vi "HFRR ADV v026 new software.vi"() -> ()   [LabVIEW 2025] (continued)
        n1473 = property on="Dashboard" class="Bool (strict)"("DisabledEnum"=w1348) -> ()  [unwired: 2 in, 2 out]
        n1474 = property on="Analysis" class="Bool (strict)"("DisabledEnum"=w1348) -> ()  [unwired: 2 in, 2 out]
        n1475 = property on="Home" class="Bool (strict)"("DisabledEnum"=w1348) -> ()  [unwired: 2 in, 2 out]
        n1476 = property on="Report" class="Bool (strict)"("DisabledEnum"=w1348) -> ()  [unwired: 2 in, 2 out]
        n1477 = property on="Calibration" class="Bool (strict)"("DisabledEnum"=w1348) -> ()  [unwired: 2 in, 2 out]
      }
      frame "About" {
        n1478 = local read "FILE"() -> (w1367:string)
        n1479 = local read "TEST FILE NAM,E SAVED"() -> (w1360:bool)
        n1480 = call <vilib>:"Trim Whitespace.vi"("string"=w1367) -> ("trimmed string"=w1366:string)  [unwired: 1 in]
        n1481 = local read "Auto Start Test"() -> (w1370:bool)
        n1482 = String Length(string=w1366) -> (length=w1365:i32)
        n1483 = Greater?(x=w1365, y=1) -> (0:w1362:bool)
        n1484 = And(x=w1362, y=w1360) -> (x .and. y?=w1361:bool)
        n1485 = local read "RUN"() -> (w1372:bool)
        n1486 = case shown="True" w1361 {
          tunnel: [T18."Disabled" ("Disabled") T18."Enabled" ("Disabled")] -> w1363
          frame False {
          }
          frame True {
          }
        }
        n1487 = Or(x=w1372, y=w1370) -> (x .or. y?=w1371:bool)
        n1488 = property on="About" class="Bool (strict)"("DisabledEnum"=T18."Enabled" ("Disabled")) -> ()  [unwired: 2 in, 2 out]
        n1489 = case shown="False" w1371 {
          tunnel: [T18."Enabled" ("Disabled") T18."Disabled" ("Disabled")] -> w1369
          frame False {
          }
          frame True {
          }
        }
        n1490 = property on="Dashboard" class="Bool (strict)"("DisabledEnum"=w1363) -> ()  [unwired: 2 in, 2 out]
        n1491 = property on="Test Setup" class="Bool (strict)"("DisabledEnum"=T18."Disabled" ("Disabled")) -> ()  [unwired: 2 in, 2 out]
        n1492 = property on="Imaging" class="Bool (strict)"("DisabledEnum"=w1369) -> ()  [unwired: 2 in, 2 out]
        n1493 = property on="Analysis" class="Bool (strict)"("DisabledEnum"=w1369) -> ()  [unwired: 2 in, 2 out]
        n1494 = property on="Home" class="Bool (strict)"("DisabledEnum"=w1369) -> ()  [unwired: 2 in, 2 out]
        n1495 = property on="Report" class="Bool (strict)"("DisabledEnum"=w1369) -> ()  [unwired: 2 in, 2 out]
      }
    }
    n1496 = local read "Quit"() -> (w1297:bool)
    "Single" <- "Single - Graph"
  }
  n1497 = disable-structure shown="Disabled" {
    disable-tunnel: [w1649 _] -> w42
    disable-tunnel: _ -> [w1648 _]
    frame Disabled {
      n1498 = while {
        tunnel: w1648 -> [_]
        tunnel: [w1650] -> w1649
        tunnel: [w1651] -> _
        i -> [w1651]
        stop <- w1650 stop-if-true
        w1667 = u16 10 items=["1.0"=10, "1.5"=15, "2.0"=20] ("stop bits (10: 1 bit)")
        n1499 = Wait (ms)(milliseconds to wait=u32 10) -> ()  [unwired: 1 out]
        n1500 = call-poly "VISA Configure Serial Port"("VISA resource name"=refnum<visa-resource-name> "ASRL1::INSTR" ("COM PORT"), "timeout (10sec)"=u32 10, "baud rate (9600)"=u32 57600, "data bits (8)"=u16 8, "stop bits (10: 1 bit)"=w1667) -> ("VISA resource name out"=w1653:refnum<visa-resource-name>, "error out"=w1662:errorcluster)  [unwired: 9 in]
        n1501 = VISA Read(VISA resource name=w1653, byte count=u32 2 ("byte count (0)")) -> (read buffer=w1661:string)  [unwired: 1 in, 3 out]
        n1502 = String Subset(string=w1661, offset (0)=0, length (rest)=2 ("length (rest)")) -> (substring=w1660:string)
        n1503 = Match Pattern(string=w1660, regular expression="<>") -> (offset past match=w1657:i32)  [unwired: 1 in, 3 out]
        n1504 = Greater Or Equal?(x=w1657, y=0) -> (x >= y?=w1652:bool)
        n1505 = case shown="True" w1652 {
          tunnel: w1653 -> [_ w1671]
          tunnel: w1662 -> [_ w1670]
          frame False {
          }
          frame True {
            n1506 = VISA Read(VISA resource name=w1671, byte count=u32 32 ("byte count (0)"), error in (no error)=w1670) -> (read buffer=w1669:string)  [unwired: 3 out]
            n1507 = String Subset(string=w1669, offset (0)=0, length (rest)=8 ("length (rest)")) -> (substring=w1673:string)
            n1508 = String Subset(string=w1669, offset (0)=8, length (rest)=8 ("length (rest)")) -> (substring=w1674:string)
            n1509 = Decimal String To Number(string=w1674) -> (number=w1681:i32)  [unwired: 2 in, 1 out]
            n1510 = Decimal String To Number(string=w1673) -> (number=w1677:i32)  [unwired: 2 in, 1 out]
            n1511 = Divide(x=w1681, y=10000) -> ()  [unwired: 1 out]
            n1512 = Divide(x=w1677, y=1000000) -> ()  [unwired: 1 out]
          }
        }
        n1513 = local read "Quit"() -> (w1650:bool)
      }
    }
    frame Enabled {
    }
  }
  n1514 = Tick Count (ms)() -> (millisecond timer value=w4:u32)
  n1515 = while {
    shift-right: [w1727] -> _
    shift-left: w6 -> [w1731]
    shift-right: [w1726] -> _
    shift-left: w5 -> [w1730]
    shift-right: [w1725] -> _
    shift-left: w6 -> [w1729]
    shift-right: [w1724] -> _
    shift-left: w5 -> [w1728]
    shift-right: [w1722] -> _
    shift-left: w4 -> [w1723]
    shift-right: [w1719] -> _
    shift-left: w3 -> [w1720]
    shift-right: [w1718] -> _
    shift-left: w3 -> [w1721]
    shift-right: [w1711] -> _
    shift-left: w3 -> [w1717]
    shift-right: [w1710] -> _
    shift-left: w3 -> [w1716]
    shift-right: [w1709] -> _
    shift-left: w3 -> [w1715]
    shift-right: [w1708] -> _
    shift-left: w3 -> [w1714]
    shift-right: [w1707] -> _
    shift-left: w3 -> [w1713]
    shift-right: [w1706] -> _
    shift-left: w3 -> [w1712]
    shift-right: [w1705] -> _
    shift-left: w3 -> [w1699]
    shift-right: [w1704] -> _
    shift-left: w3 -> [w1698]
    shift-right: [w1703] -> _
    shift-left: w3 -> [w1697]
    shift-right: [w1702] -> _
    shift-left: w3 -> [w1696]
    shift-right: [w1701] -> _
    shift-left: w3 -> [w1695]
    shift-right: [w1700] -> _
    shift-left: w3 -> [w1694]
    shift-right: [w1685] -> _
    shift-left: w3 -> [w1688]
    shift-right: [w1684] -> _
    shift-left: w3 -> [w1687]
    shift-right: [w1683] -> _
    shift-left: w3 -> [w1686]
    stop <- w1733 stop-if-true
    n1516 = local read "Read UNO"() -> (w1692:string)
    n1517 = local read "Error  2"() -> (w1732:errorcluster)
    n1518 = String Length(string=w1692) -> (length=w1691:i32)
    n1519 = call <vilib>:"Trim Whitespace.vi"("string"=w1692) -> ("trimmed string"=w1693:string)  [unwired: 1 in]
    n1520 = Greater Or Equal?(x=w1691, y=23) -> (x >= y?=w1689:bool)
    n1521 = case shown="No Error" w1732 {
      tunnel: w1731 -> [w1779 w1875]
      tunnel: w1730 -> [w1778 w1874]
      tunnel: w1729 -> [w1777 w1873]
      tunnel: w1728 -> [w1776 w1872]
      tunnel: [w1775 w1875] -> w1727
      tunnel: [w1774 w1874] -> w1726
      tunnel: [w1773 w1873] -> w1725
      tunnel: [w1772 w1872] -> w1724
      tunnel: w1723 -> [w1771 w1871]
      tunnel: [w1770 w1871] -> w1722
      tunnel: w1720 -> [w1769 w1870]
      tunnel: w1721 -> [w1768 w1869]
      tunnel: [w1767 w1870] -> w1719
      tunnel: [w1766 w1869] -> w1718
      tunnel: w1717 -> [w1765 w1868]
      tunnel: w1716 -> [w1764 w1867]
      tunnel: w1715 -> [w1763 w1866]
      tunnel: w1714 -> [w1762 w1865]
      tunnel: w1713 -> [w1761 w1864]
      tunnel: w1712 -> [w1760 w1863]
      tunnel: [w1759 w1868] -> w1711
      tunnel: [w1758 w1867] -> w1710
      tunnel: [w1757 w1866] -> w1709
      tunnel: [w1756 w1865] -> w1708
      tunnel: [w1755 w1864] -> w1707
      tunnel: [w1754 w1863] -> w1706
      tunnel: w1699 -> [w1753 w1862]
      tunnel: [w1752 w1862] -> w1705
      tunnel: [w1751 w1858] -> w1704
      tunnel: [w1750 w1857] -> w1703
      tunnel: [w1749 w1861] -> w1702
      tunnel: [w1748 w1860] -> w1701
      tunnel: [w1747 w1859] -> w1700
      tunnel: w1698 -> [w1746 w1861]
      tunnel: w1697 -> [w1745 w1860]
      tunnel: w1696 -> [w1744 w1859]
      tunnel: w1695 -> [w1743 w1858]
      tunnel: w1694 -> [w1742 w1857]
      tunnel: w1693 -> [w1741 _]
      tunnel: w1689 -> [w1740 _]
      tunnel: w1688 -> [w1739 w1856]
      tunnel: w1687 -> [w1738 w1855]
      tunnel: w1686 -> [w1737 w1854]
      tunnel: [w1736 w1856] -> w1685
      tunnel: [w1735 w1855] -> w1684
      tunnel: [w1734 w1854] -> w1683
      frame No Error {
        n1522 = case shown="True" w1740 {
          tunnel: w1779 -> [w1795 w1847]
          tunnel: w1778 -> [w1794 w1846]
          tunnel: w1777 -> [w1793 w1845]
          tunnel: w1776 -> [w1792 w1844]
          tunnel: [w1795 w1843] -> w1775
          tunnel: [w1794 w1842] -> w1774
          tunnel: [w1793 w1841] -> w1773
          tunnel: [w1792 w1840] -> w1772
          tunnel: w1771 -> [w1791 w1838]
          tunnel: [w1791 w1837] -> w1770
          tunnel: w1769 -> [w1790 w1836]
          tunnel: w1768 -> [w1789 w1835]
          tunnel: [w1790 w1834] -> w1767
          tunnel: [w1789 w1833] -> w1766
          tunnel: w1765 -> [w1788 w1832]
          tunnel: w1764 -> [w1787 w1831]
          tunnel: w1763 -> [w1786 w1830]
          tunnel: w1762 -> [w1785 w1829]
          tunnel: w1761 -> [w1784 w1828]
          tunnel: w1760 -> [w1783 w1827]
          tunnel: [w1788 w1826] -> w1759
          tunnel: [w1787 w1825] -> w1758
          tunnel: [w1786 w1824] -> w1757
          tunnel: [w1785 w1823] -> w1756
          tunnel: [w1784 w1822] -> w1755
          tunnel: [w1783 w1821] -> w1754
          tunnel: w1753 -> [w1801 w1820]
          tunnel: [w1801 w1819] -> w1752
          tunnel: [w1798 w1818] -> w1751
          tunnel: [w1797 w1817] -> w1750
          tunnel: [w1800 w1816] -> w1749
          tunnel: [w1796 w1815] -> w1748
          tunnel: [w1799 w1814] -> w1747
          tunnel: w1746 -> [w1800 w1813]
          tunnel: w1745 -> [w1799 w1812]
          tunnel: w1744 -> [w1798 w1811]
          tunnel: w1743 -> [w1797 w1810]
          tunnel: w1742 -> [w1796 w1809]
          tunnel: w1741 -> [_ w1808]
          tunnel: w1739 -> [w1782 w1807]
          tunnel: w1738 -> [w1781 w1806]
          tunnel: w1737 -> [w1780 w1805]
          tunnel: [w1782 w1804] -> w1736
          tunnel: [w1781 w1803] -> w1735
          tunnel: [w1780 w1802] -> w1734
          frame False {
          }
          frame True {
            n1523 = Tick Count (ms)() -> (millisecond timer value=w1839:u32)
            n1524 = String To Byte Array(string=w1808) -> (unsigned byte array=w1852:u8[])
            n1525 = Array Size(array=w1852) -> (size(s)=w1851:i32)
            n1526 = formula code="// --- INTERNAL VARIABLE DECLARATIONS ---\nint i = 0;\nint k = 0;\nint start_idx = -1;\nint end_idx = -1;\nint phase = 0;\nint sign0 = 1;\nint sign1 = 1;\nint ch0_val = 0;   \nint ch1_val = 0;   \nfloat ch0_raw = 0.0;\nfloat ch1_raw = 0.0;\nfloat temp0 = 0.0;\nfloat temp1 = 0.0;\nfloat ch0_clean = 0.0;\nfloat ch1_clean = 0.0;\n\n// Temporal intermediate variables for calculation smoothing\nfloat raw_p2p_v = 0.0;\nfloat raw_friction = 0.0;\nfloat raw_cof = 0.0;\n\n// Initialize output variables to current shift register states right away\nout_LVDT_Min_V = in_LVDT_Min_V;\nout_LVDT_Max_V = in_LVDT_Max_V;\nout_LVDT_P2P_V = in_LVDT_P2P_V;\nout_Piezo_P2P = in_Piezo_P2P;\nout_Friction_N = in_Friction_N;\nout_COF = in_COF;\nwindow_ready = 0;\n\n// --- STEP 1: PARSE EVERY STRING IN THE BYTE ARRAY ---\nif (array_size > 2) {\n    for (i = 0; i < array_size - 1; i++) {\n        if (raw_bytes[i] == 42) { // '*' character detected\n            start_idx = i;\n        }\n        \n        // Match standard delimiter sequence \";&\" or end window character\n        if (raw_bytes[i] == 59 && raw_bytes[i+1] == 38 && start_idx != -1) { \n            end_idx = i;\n            ch0_val = 0;\n            ch1_val = 0;\n            sign0 = 1;\n            sign1 = 1;\n            phase = 0; \n\n            for (k = start_idx + 1; k < end_idx; k++) {\n                if (raw_bytes[k] == 45) { // '-' sign\n                    if (phase == 0) sign0 = -1;\n                    else sign1 = -1;\n                }\n                else if (raw_bytes[k] == 43) { // '+' sign\n                    if (phase == 0) sign0 = 1;\n                    else sign1 = 1;\n                }\n                else if (raw_bytes[k] == 59) { // ';' delimiter\n                    phase = 1; \n                }\n                else if (raw_bytes[k] >= 48 && raw_bytes[k] <= 57) { // Numeric ASCII digits\n                    if (phase == 0) {\n                        ch0_val = (ch0_val * 10) + (raw_bytes[k] - 48);\n                    } else {\n                        ch1_val = (ch1_val * 10) + (raw_bytes[k] - 48);\n                    }\n                }\n            }\n\n            // Implicit type conversion\n            ch0_raw = ch0_val * sign0 * 1.0;\n            ch1_raw = ch1_val * sign1 * 1.0;\n\n            // --- STEP 2: 3-SAMPLE MEDIAN FILTER ---\n            m0_2 = m0_1; m0_1 = m0_0; m0_0 = ch0_raw;\n            float s0_0 = m0_0; float s0_1 = m0_1; float s0_2 = m0_2;\n            if (s0_0 > s0_1) { temp0 = s0_0; s0_0 = s0_1; s0_1 = temp0; }\n            if (s0_1 > s0_2) { temp0 = s0_1; s0_1 = s0_2; s0_2 = temp0; }\n            if (s0_0 > s0_1) { temp0 = s0_0; s0_0 = s0_1; s0_1 = temp0; }\n            ch0_clean = s0_1;\n\n            m1_2 = m1_1; m1_1 = m1_0; m1_0 = ch1_raw;\n            float s1_0 = m1_0; float s1_1 = m1_1; float s1_2 = m1_2;\n            if (s1_0 > s1_1) { temp1 = s1_0; s1_0 = s1_1; s1_1 = temp1; }\n            if (s1_1 > s1_2) { temp1 = s1_1; s1_1 = s1_2; s1_2 = temp1; }\n            if (s1_0 > s1_1) { temp1 = s1_0; s1_0 = s1_1; s1_1 = temp1; }\n            ch1_clean = s1_1;\n\n            // --- STEP 3: EXPONENTIAL FILTER (STREAM LEVEL) ---\n            if (ch0_filt == 0.0) ch0_filt = ch0_clean;\n            if (ch1_filt == 0.0) ch1_filt = ch1_clean;\n\n            ch0_filt = ch0_filt + (ch0_clean - ch0_filt) * 0.125;\n            ch1_filt = ch1_filt + (ch1_clean - ch1_filt) * 0.125;\n\n            // --- STEP 4: MIN/MAX WINDOW CONTINUOUS ACCUMULATION ---\n            if (ch0_filt > max_ch0) max_ch0 = ch0_filt;\n            if (ch0_filt < min_ch0) min_ch0 = ch0_filt;\n            if (ch1_filt > max_ch1) max_ch1 = ch1_filt;\n            if (ch1_filt < min_ch1) min_ch1 = ch1_filt;\n\n            start_idx = -1; \n        }\n    }\n}\n\n// --- STEP 5: WINDOW EVALUATION ENGINE ---\nif (((current_time_ms - start_time_ms) >= 50) && (min_ch0 < 9000000.0) && (max_ch0 > -9000000.0)) {\n    window_ready = 1;\n\n    // Linear Bit-to-Voltage Transformations\n    out_LVDT_Min_V = (min_ch0 * VREF) / 8388607.0;\n    out_LVDT_Max_V = (max_ch0 * VREF) / 8388607.0;\n    raw_p2p_v = out_LVDT_Max_V - out_LVDT_Min_V;\n\n    // Piezo scaling calculations\n    out_Piezo_P2P = max_ch1 - min_ch1;\n    raw_friction = out_Piezo_P2P * PIEZO_CAL_FACTOR;\n    raw_cof = raw_friction / NORMAL_FORCE;\n\n    // --- STEP 6: OUTPUT METRIC SMOOTHING (Low-Pass Filter Alpha = 0.20) ---\n    // Seed initial historical metrics if first loop iteration\n    if (hist_LVDT_P2P == 0.0) hist_LVDT_P2P = raw_p2p_v;\n    if (hist_Friction == 0.0) hist_Friction = raw_friction;\n    if (hist_COF == 0.0)      hist_COF = raw_cof;\n\n    // Apply exponential output dampening\n    hist_LVDT_P2P = hist_LVDT_P2P + (raw_p2p_v - hist_LVDT_P2P) * 0.05;\n    hist_Friction = hist_Friction + (raw_friction - hist_Friction) * 0.05;\n    hist_COF      = hist_COF + (raw_cof - hist_COF) * 0.05;\n\n    // Direct smoothed parameters out to UI Indicators\n    out_LVDT_P2P_V = hist_LVDT_P2P;\n    out_Friction_N = hist_Friction;\n    out_COF        = hist_COF;\n\n    // Reset tracking targets to extreme boundaries safely\n    min_ch0 = 9999999.0;\n    max_ch0 = -9999999.0;\n    min_ch1 = 9999999.0;\n    max_ch1 = -9999999.0;\n\n    start_time_ms = current_time_ms;\n}"("raw_bytes"=w1852, "array_size"=w1851, "VREF"="VREF", "PIEZO_CAL_FACTOR"="PIEZO_CAL_FACTOR", "NORMAL_FORCE"="NORMAL_FORCE", "min_ch0"=w1847, "max_ch0"=w1846, "min_ch1"=w1845, "max_ch1"=w1844, "current_time_ms"=w1839, "start_time_ms"=w1838, "ch0_filt"=w1836, "ch1_filt"=w1835, "m0_0"=w1832, "m0_1"=w1831, "m0_2"=w1830, "m1_0"=w1829, "m1_1"=w1828, "m1_2"=w1827, "in_LVDT_Min_V"=w1820, "in_LVDT_Max_V"=w1813, "in_LVDT_P2P_V"=w1812, "in_Piezo_P2P"=w1811, "in_Friction_N"=w1810, "in_COF"=w1809, "hist_LVDT_P2P"=w1807, "hist_Friction"=w1806, "hist_COF"=w1805) -> ("window_ready"=→"Valid_data":dbl, "out_LVDT_Min_V"=w1819:dbl, "out_LVDT_Max_V"=w1818:dbl, "out_LVDT_P2P_V"=w1817:dbl, "out_Piezo_P2P"=w1816:dbl, "out_Friction_N"=w1815:dbl, "out_COF"=w1814:dbl, "min_ch0"=w1843:dbl, "max_ch0"=w1842:dbl, "min_ch1"=w1841:dbl, "max_ch1"=w1840:dbl, "start_time_ms"=w1837:u32, "ch0_filt"=w1834:dbl, "ch1_filt"=w1833:dbl, "m0_0"=w1826:dbl, "m0_1"=w1825:dbl, "m0_2"=w1824:dbl, "m1_0"=w1823:dbl, "m1_1"=w1822:dbl, "m1_2"=w1821:dbl, "hist_LVDT_P2P"=w1804:dbl, "hist_Friction"=w1803:dbl, "hist_COF"=w1802:dbl)
            "LVDT MIN" <- w1819
            "LVDT MAX" <- w1818
            "LVDT Peak" <- w1817
            "pizo raw" <- w1816
            "Friction" <- w1815
            "cof" <- w1814
          }
        }
      }
      frame Error {
      }
    }
    n1527 = local read "Quit"() -> (w1733:bool)
  }
  n1528 = disable-structure shown="Disabled" {
    disable-tunnel: errorcluster {"status"=TRUE, "code"=0, "source"="Init"} ("error IO") -> [w1878 _]
    disable-tunnel: [w1876 _] -> w45
    frame Disabled {
      n1529 = while {
        shift-right: [w1894] -> w1880
        shift-left: _ -> [w1885]
        shift-right: [w1893] -> w1879
        shift-left: w1878 -> [w1887]
        tunnel: [w1882] -> w1876
        tunnel: [w1892] -> _
        i -> [w1892]
        stop <- w1882 stop-if-true
        n1530 = local read "Port 1a"() -> (w1888:bool)
        n1531 = local read "Port 3"() -> (w1889:bool)
        n1532 = local read "Com Port 1"() -> (w1886:refnum<visa-resource-name>)
        n1533 = Or(x=w1889, y=w1888) -> (x .or. y?=w1891:bool)
        n1534 = Unbundle(w1887) -> ("status"=→"Port 3":bool)  [unwired: 2 out]
        n1535 = Not Equal?(x=w1886, y=w1885) -> (x != y?=w1883:bool)
        n1536 = case shown="True" w1891 {
          frame False {
            w1897 = TRUE ("Visible")
            n1537 = property on="Port 1a" class="Bool (strict)"("Visible"=w1897) -> ()  [unwired: 2 in, 2 out]
            n1538 = property on="Port 3" class="Bool (strict)"("Visible"=w1897) -> ()  [unwired: 2 in, 2 out]
          }
          frame True {
            w1898 = TRUE ("Visible")
            n1539 = property on="Port 1a" class="Bool (strict)"("Visible"=w1898) -> ()  [unwired: 2 in, 2 out]
            n1540 = property on="Port 3" class="Bool (strict)"("Visible"=w1898) -> ()  [unwired: 2 in, 2 out]
          }
        }
        n1541 = Wait (ms)(milliseconds to wait=u32 40) -> ()  [unwired: 1 out]
        n1542 = case shown="True" w1883 {
          tunnel: [w1895 errorcluster {"status"=TRUE, "code"=0, "source"="Init"} ("error out")] -> w1884
          tunnel: w1887 -> [w1895 _]
          frame False {
          }
          frame True {
          }
        }
        n1543 = case shown="Error" w1884 {
          selector: w1884 -> [w1905 w1923]
          tunnel: [w1908 w1927] -> w1894
          tunnel: [w1907 w1921] -> w1893
          tunnel: w1885 -> [w1906 w1925]
          frame No Error {
            n1544 = property class="Instr"(reference=w1906, error in=w1905) -> (reference out=w1903:refnum<visa-resource-name>, error out=w1904:errorcluster, "Serial Settings:Number of Bytes at Serial Port"=w1900:u32)
            n1545 = Greater?(x=w1900, y=u32 5) -> (0:w1899:bool)
            n1546 = Not(x=w1899) -> (.not. x?=→"Port 1a":bool)
            n1547 = while {
              tunnel: [w1916] -> w1907
              tunnel: [w1915] -> w1908
              tunnel: w1904 -> [w1914]
              tunnel: w1903 -> [w1913]
              stop <- TRUE stop-if-true
              n1548 = property class="Instr" props=["Serial Settings:Number of Bytes at Serial Port"](reference=w1913, error in=w1914) -> (reference out=w1918:refnum<visa-resource-name>, error out=w1917:errorcluster)  [unwired: 1 out]
              n1549 = VISA Read(VISA resource name=w1918, byte count=u32 50, error in (no error)=w1917) -> (VISA resource name out=w1915:refnum<visa-resource-name>, read buffer=w1910:string, error out=w1916:errorcluster)  [unwired: 1 out]
              n1550 = Wait (ms)(milliseconds to wait=u32 5) -> ()  [unwired: 1 out]
            }
          }
          frame Error {
            w1933 = u16 0 items=["None", "XON/XOFF", "RTS/CTS", "XON/XOFF & RTS/CTS", "DTR/DSR", "XON/XOFF & DTR/DSR"] ("flow control (0:none)  2")
            w1931 = u16 10 items=["1.0"=10, "1.5"=15, "2.0"=20] ("stop bits 2")
            w1929 = u16 0 items=["None", "Odd", "Even", "Mark", "Space"] ("parity 2")
            w1930 = u32 10000  # timeout (10sec)
            n1551 = VISA Close(VISA resource name=w1925, error in (no error)=w1923) -> (error out=w1926:errorcluster)
            n1552 = local write "Port 1a"(FALSE ("Port 1a")) -> ()
            n1553 = local read "Com Port 1"() -> (w1920:refnum<visa-resource-name>)
            n1554 = call <vilib>:"Clear Errors.vi"("error in (no error)"=w1926) -> ("error out"=w1924:errorcluster)  [unwired: 5 in, 1 out]
            n1555 = call-poly "VISA Configure Serial Port"("VISA resource name"=w1920, "timeout (10sec)"=w1930, "baud rate (9600)"=u32 250000 ("baud rate  2"), "data bits (8)"=u16 8 ("data bits  2"), "parity (0:none)"=w1929, "error in (no error)"=w1924, "stop bits (10: 1 bit)"=w1931, "flow control (0:none)"=w1933) -> ("VISA resource name out"=w1934:refnum<visa-resource-name>, "error out"=w1935:errorcluster)  [unwired: 6 in]
            n1556 = flat-sequence {
              tunnel: w1934 -> [w1937]
              tunnel: w1935 -> [w1936]
              tunnel: [w1937] -> w1927
              tunnel: [w1936] -> w1921
              frame #0 {
                n1557 = Wait (ms)(milliseconds to wait=u32 50) -> ()  [unwired: 1 out]
              }
            }
            "Residual Uno" <- ""
          }
        }
        n1558 = local read "Quit"() -> (w1882:bool)
        "Error Uno" <- w1887
      }
      n1559 = VISA Close(VISA resource name=w1880, error in (no error)=w1879) -> (error out=w1877:errorcluster)
      n1560 = call <vilib>:"Clear Errors.vi"("error in (no error)"=w1877) -> ()  [unwired: 5 in, 2 out]
    }
    frame Enabled {
    }
  }
  n1561 = while {
    stop <- w1948 stop-if-true
    # "V0OLTAGE TO STROKE (peice vise calibration)"
    n1562 = local read "LVDT MIN"() -> (w1940:dbl)
    n1563 = local read "LVDT Peak"() -> (w1939:dbl)
    n1564 = Wait (ms)(milliseconds to wait=u32 10) -> ()  [unwired: 1 out]
    n1565 = formula code="// Dynamic Parameterized Linear Interpolation Node\n// Inputs: vpp_val, voltages (Array), distances (Array)\n// Outputs: stroke\n\nint i = 0;\nint segments = 11; // 12 points make 11 interpolation segments\n\n// 1. Lower Boundary Clamp\nif (vpp_val <= voltages[0]) {\n    stroke = distances[0];\n}\n// 2. Upper Boundary Clamp\nelse if (vpp_val >= voltages[segments]) {\n    stroke = distances[segments];\n}\n// 3. Dynamic Segment Search Loop\nelse {\n    stroke = distances[0]; // Fallback baseline\n    for (i = 0; i < segments; i++) {\n        if (vpp_val >= voltages[i] && vpp_val <= voltages[i+1]) {\n            // Standard linear interpolation formula using array lookups\n            stroke = distances[i] + (vpp_val - voltages[i]) * (distances[i+1] - distances[i]) / (voltages[i+1] - voltages[i]);\n            break; // Segment found, safely exit the loop\n        }\n    }\n}"("vpp_val"=w1939, "voltages"="calibration values", "distances"="STROKE") -> ("stroke"=→"LVDT STROKE":dbl)
    n1566 = local read "Calibration Tare Value"() -> (w1944:dbl)
    n1567 = local read "Calibration Tare"() -> (w1942:bool)
    n1568 = Subtract(x=w1940, y=w1944) -> (x-y=→"LVDT STROKE  Calibration":dbl)
    n1569 = case shown="True" w1942 {
      selector: w1942 -> [_ w1950]
      tunnel: w1940 -> [_ w1951]
      frame False {
      }
      frame True {
        n1570 = Not(x=w1950) -> (.not. x?=w1949:bool)
        n1571 = local write "Calibration Tare"(w1949) -> ()
        "Calibration Tare Value" <- w1951
      }
    }
    n1572 = local read "Quit"() -> (w1948:bool)
  }
  n1573 = while {
    stop <- w1971 stop-if-true
    n1574 = call <vilib>:"High Resolution Polling Wait.vi"("seconds to wait"=0.02) -> ()  [unwired: 10 in, 1 out]
    n1575 = local read "Due read"() -> (w1969:string)
    n1576 = Spreadsheet String To Array(delimiter (Tab)=";", format string="", spreadsheet string=w1969, array type (2D Dbl)=string[] []) -> (array=w1966:string[])
    n1577 = Fract/Exp String To Number(string=w1966) -> (number=w1965:dbl[])  [unwired: 3 in, 1 out]
    n1578 = Index Array(array=w1965) -> (element #1=→"Sample Temperature":dbl, element #2=→"Target Sample Temperature":dbl, element #3=→"Current Duty Cycle":dbl, element #4=→"Ambient Temperature":dbl, element #5=→"Dac Status":dbl, element #6=→"Vpp":dbl, element #7=→"Active Error Code":dbl, element #8=→"Kp":dbl, element #9=→"Ki":dbl, element #10=→"Kd":dbl, element #11=→"SampleRaw":dbl, element #12=→"AmbRaw":dbl)  [unwired: 12 in]
    n1579 = local read "Quit"() -> (w1971:bool)
  }
  n1580 = while {
    shift-right: [w1985] -> w41
    shift-left: _ -> [w1977]
    shift-right: [w1972] -> w40
    shift-left: errorcluster {"status"=FALSE, "code"=0, "source"="Init"} ("error out") -> [w1979]
    tunnel: [w1974] -> w44
    tunnel: [w1984] -> _
    i -> [w1984]
    stop <- w1974 stop-if-true
    n1581 = local read "Com Port 2"() -> (w1978:refnum<visa-resource-name>)
    n1582 = local read "Port 2a"() -> (w1980:bool)
    n1583 = Unbundle(w1979) -> ("status"=→"Port 4":bool)  [unwired: 2 out]
    n1584 = call <vilib>:"High Resolution Polling Wait.vi"("seconds to wait"=0.02) -> ()  [unwired: 10 in, 1 out]
    n1585 = local read "Port 4"() -> (w1981:bool)
    n1586 = Not Equal?(x=w1978, y=w1977) -> (x != y?=w1976:bool)
    n1587 = Or(x=w1981, y=w1980) -> (x .or. y?=w1983:bool)
    n1588 = case shown="False" w1983 {
      frame False {
        w1988 = TRUE ("Visible")
        n1589 = property on="Port 2a" class="Bool (strict)"("Visible"=w1988) -> ()  [unwired: 2 in, 2 out]
        n1590 = property on="Port 4" class="Bool (strict)"("Visible"=w1988) -> ()  [unwired: 2 in, 2 out]
      }
      frame True {
        w1989 = TRUE ("Visible")
        n1591 = property on="Port 2a" class="Bool (strict)"("Visible"=w1989) -> ()  [unwired: 2 in, 2 out]
        n1592 = property on="Port 4" class="Bool (strict)"("Visible"=w1989) -> ()  [unwired: 2 in, 2 out]
      }
    }
    n1593 = case shown="True" w1976 {
      tunnel: [w1986 errorcluster {"status"=TRUE, "code"=0, "source"="Init"} ("error out")] -> w1975
      tunnel: w1979 -> [w1986 _]
      frame False {
      }
      frame True {
      }
    }
    n1594 = case shown="No Error" w1975 {
      selector: w1975 -> [w2002 w2033]
      tunnel: [w1995 w2038] -> w1985
      tunnel: [w2003 w2031] -> w1972
      tunnel: w1977 -> [w2004 w2036]
      frame No Error {
        n1595 = property class="Instr" props=["Serial Settings:Number of Bytes at Serial Port"](reference=w2004, error in=w2002) -> (reference out=w1996:refnum<visa-resource-name>, error out=w2001:errorcluster)  [unwired: 1 out]
        n1596 = while {
          tunnel: [w2012] -> w1997
          tunnel: [w2011] -> w1998
          tunnel: w2001 -> [w2010]
          tunnel: w1996 -> [w2009]
          tunnel: [w2008] -> _
          i -> [w2008]
          stop <- TRUE stop-if-true
          n1597 = property class="Instr" props=["Serial Settings:Number of Bytes at Serial Port"](reference=w2009, error in=w2010) -> (reference out=w2014:refnum<visa-resource-name>, error out=w2013:errorcluster)  [unwired: 1 out]
          n1598 = VISA Read(VISA resource name=w2014, byte count=u32 1000, error in (no error)=w2013) -> (VISA resource name out=w2011:refnum<visa-resource-name>, read buffer=→"Due read":string, error out=w2012:errorcluster)  [unwired: 1 out]
        }
        n1599 = local read "Due Write"() -> (w1994:string)
        n1600 = call <vilib>:"Trim Whitespace.vi"("string"=w1994) -> ("trimmed string"=w1993:string)  [unwired: 1 in]
        n1601 = Not Equal?(x=w1993, y="") -> (x != y?=w1999:bool)
        n1602 = VISA Flush I/O Buffer(VISA resource name=w1998) -> (VISA resource name out=w1991:refnum<visa-resource-name>, error out=→"error out 10":errorcluster)  [unwired: 2 in]
        n1603 = case shown="True" w1999 {
          tunnel: w1991 -> [w2016 w2021]
          tunnel: [w2016 w2025] -> w1995
          tunnel: w1997 -> [w2015 w2020]
          tunnel: [w2015 w2023] -> w2003
          tunnel: w1993 -> [_ w2019]
          tunnel: [_ w2022] -> _
          frame False {
            # "DATA  WRITE LOOP"
          }
          frame True {
            n1604 = Concatenate Strings(w2019, "\r\n") -> (w2018:string)
            n1605 = VISA Write(VISA resource name=w2021, write buffer=w2018, error in (no error)=w2020) -> (VISA resource name out=w2025:refnum<visa-resource-name>, return count=w2022:u32, error out=w2024:errorcluster)
            n1606 = flat-sequence {
              tunnel: w2024 -> [w2027]
              tunnel: [w2027] -> w2023
              frame #0 {
                n1607 = local write "Due Write"("" ("Command")) -> ()
                n1608 = Wait (ms)(milliseconds to wait=u32 5) -> ()  [unwired: 1 out]
              }
            }
          }
        }
        "Port 2a" <- TRUE ("Port 2a")
      }
      frame Error {
        w2044 = u16 0 items=["None", "XON/XOFF", "RTS/CTS", "XON/XOFF & RTS/CTS", "DTR/DSR", "XON/XOFF & DTR/DSR"] ("flow control (0:none)  2")
        w2042 = u16 10 items=["1.0"=10, "1.5"=15, "2.0"=20] ("stop bits 2")
        w2040 = u16 0 items=["None", "Odd", "Even", "Mark", "Space"] ("parity 2")
        w2041 = u32 10000  # timeout (10sec)
        n1609 = VISA Clear(VISA resource name=w2036, error in (no error)=w2033) -> (VISA resource name out=w2035:refnum<visa-resource-name>, error out=w2034:errorcluster)
        n1610 = VISA Close(VISA resource name=w2035, error in (no error)=w2034) -> (error out=w2037:errorcluster)
        n1611 = call <vilib>:"Clear Errors.vi"("error in (no error)"=w2037) -> ()  [unwired: 5 in, 2 out]
        n1612 = local write "Port 2a"(FALSE ("Port 2a")) -> ()
        n1613 = local read "Com Port 2"() -> (w2030:refnum<visa-resource-name>)
        "visa due" <- w2030
        n1614 = call-poly "VISA Configure Serial Port"("VISA resource name"=w2030, "timeout (10sec)"=w2041, "baud rate (9600)"=u32 250000 ("baud rate  2"), "data bits (8)"=u16 8 ("data bits  2"), "parity (0:none)"=w2040, "stop bits (10: 1 bit)"=w2042, "flow control (0:none)"=w2044) -> ("VISA resource name out"=w2045:refnum<visa-resource-name>, "error out"=w2046:errorcluster)  [unwired: 7 in]
        n1615 = flat-sequence {
          tunnel: w2045 -> [w2048]
          tunnel: w2046 -> [w2047]
          tunnel: [w2048] -> w2038
          tunnel: [w2047] -> w2031
          frame #0 {
            n1616 = Wait (ms)(milliseconds to wait=u32 50) -> ()  [unwired: 1 out]
          }
        }
        "Residual Due" <- ""
      }
    }
    "error out 9" <- w1972
    n1617 = local read "Quit"() -> (w1974:bool)
    "Error Due" <- w1979
  }
  n1618 = local write "FRICVALZ"(0.0 ("FRICVALZ")) -> ()
  n1619 = property on="RUN" class="Bool (strict)"("Visible"=TRUE) -> ()  [unwired: 2 in, 2 out]
  n1620 = while {
    tunnel: [w2063] -> _
    tunnel: [w2050] -> w54
    i -> [w2063]
    stop <- w2050 stop-if-true
    n1621 = local read "conststatus"() -> (w2054:dbl)
    n1622 = local read "Main Tab"() -> (w2052:T2)
    n1623 = local read "EDIT"() -> (w2069:bool)
    n1624 = local read "Rate"() -> (w2068:dbl)
    n1625 = case shown="True" w2069 {
      tunnel: [FALSE TRUE] -> _
      frame False {
      }
      frame True {
      }
    }
    n1626 = Equal?(x=w2052, y=T26."About" ("Main Tab")) -> (x = y?=w2061:bool)
    n1627 = Equal?(x=w2054, y=0.0) -> (x = y?=w2055:bool)
    n1628 = Divide(x=1.0, y=w2068) -> (x/y=w2064:dbl)
    "Time 2" <- w2064
    n1629 = case shown="True" w2055 {
      frame False {
      }
      frame True {
        # "C:\\WinDucom\\calibrate WO 2391.dcf"
        n1630 = local write "Lan flag"(22) -> ()
        n1631 = local write "conststatus"(10.0 ("rpm value : 2")) -> ()
        n1632 = String To Path(string="C:\\LAB-IQ\\calibrate WO 2465.dcf") -> (path=w2075:path)
        n1633 = Open/Create/Replace File "Open File"(file path (use dialog)=w2075) -> (refnum out=w2073:refnum<file>)  [unwired: 5 in, 2 out]
        n1634 = for {
          N: 23 -> [_]
          tunnel: w2073 -> [w2084]
          i -> [w2078]
          (unwired) TRUE ("line mode (F)")
          n1635 = Read from Text File "Read File"(file (use dialog)=w2084) -> (text=w2083:string)  [unwired: 3 in, 3 out]
          n1636 = Match Pattern(string=w2083, regular expression="]") -> (after substring=w2081:string)  [unwired: 1 in, 3 out]
          n1637 = String Subset(string=w2083, offset (0)=5, length (rest)=10 ("length (rest)")) -> (substring=w2076:string)
          n1638 = Fract/Exp String To Number(string=w2076) -> (number=w2077:dbl)  [unwired: 3 in, 1 out]
          n1639 = Match Pattern(string=w2081, regular expression="-") -> (before substring=w2079:string)  [unwired: 1 in, 3 out]
          n1640 = case shown="10" w2078 {
            tunnel: w2077 -> [_ _ _ _ _ _ _ _ _ _ w2091 _ _ _ _ _ _ _ _ _ _ _ _ _]
            tunnel: w2079 -> [_ _ _ _ w2087 w2088 w2089 _ _ _ _ _ _ _ _ _ _ _ _ _ w2092 w2093 w2094 _]
            frame 0 {
            }
            frame 1 {
            }
            frame 2 {
            }
            frame 3 {
            }
            frame 4 {
              n1641 = local write "Com Port 1"(w2087) -> ()
            }
            frame 5 {
              n1642 = local write "Com Port 2"(w2088) -> ()
              n1643 = local write "visa due"(w2088) -> ()
            }
            frame 6 {
              n1644 = String To Path(string=w2089) -> (path=w2090:path)
              n1645 = local write "File Path"(w2090) -> ()
              "String" <- w2089
            }
            frame 7 {
            }
            frame 8 {
            }
            frame 9 {
            }
            frame 10 {
              n1646 = local write "Language Selection"(w2091) -> ()
            }
            frame 11 {
            }
            frame 12 {
            }
            frame 13 {
            }
            frame 14 {
            }
            frame 15 {
            }
            frame 16 {
            }
            frame 17 {
            }
            frame 18 {
            }
            frame 21 {
            }
            frame 22 {
              n1647 = local write "Com Port 3"(w2092) -> ()
            }
            frame 20 {
              n1648 = local write "Camera Port :"(w2093) -> ()
            }
            frame 19 {
              n1649 = local write "C3 :"(w2094) -> ()
            }
            frame 23, Default {
            }
          }
        }
      }
    }
    n1650 = Select(t=u32 2500 ("milliseconds to wait"), s=w2061, f=u32 500 ("milliseconds to wait")) -> (s? t:f=w2059:u32)
    n1651 = Multiply(x=w2064, y=w2059) -> (x*y=w2066:dbl)
    n1652 = call "Elapsed Time2"("Time Target (s)"=w2066, "Auto Reset"=TRUE) -> ("Time has Elapsed"=w2056:bool)  [unwired: 10 in, 7 out]
    n1653 = case shown="True" w2056 {
      frame False {
      }
      frame True {
        n1654 = stacked-sequence {
          frame #0 {
            # "DATA PROCESSING"
            # "115 mV/N"
            n1655 = local read "Sample Temperature"() -> (w2097:dbl)
            n1656 = local read "RH Numeric:"() -> (→"Humidity ( %RH )" →"Hum" →"Hum 2":dbl)
            n1657 = local read "FRICVALZ"() -> (w2114:dbl)
            n1658 = local read "Friction"() -> (w2100:dbl)
            n1659 = call <vilib>:"Mean PtByPt.vi"("x"=w2097, "sample length"=100) -> ("mean"=w2096:dbl)  [unwired: 2 in, 1 out]
            "TEMP 2" <- w2096
            "TEMP 3" <- w2096
            n1660 = Subtract(x=w2100, y=w2114) -> (x-y=w2109:dbl)
            "FF 2" <- w2109
            "FF 4" <- w2109
            n1661 = local read "Ambient Temperature"() -> (→"AIR TEMP":dbl)
            n1662 = local read "TEMP"() -> (w2113:dbl)
            n1663 = local write "FF 3"(w2109) -> ()
            n1664 = Compound Arithmetic op=OR("FRICVALZ 4", "FRICVALZ 3", "FRICVALZ 2") -> (w2105:bool)
            n1665 = case shown="True" w2105 {
              tunnel: w2100 -> [_ w2120]
              frame False {
              }
              frame True {
                w2119 = FALSE ("FRICVALZ")
                n1666 = local write "FRICVALZ 3"(w2119) -> ()
                n1667 = local write "FRICVALZ 2"(w2119) -> ()
                n1668 = local write "FRICVALZ 4"(w2119) -> ()
                "FRICVALZ" <- w2120
              }
            }
            n1669 = Not A Number/Path/Refnum?(number/path/refnum=w2113) -> (NaN/Path/Refnum?=w2112:bool)
            n1670 = Not A Number/Path/Refnum?(number/path/refnum=w2109) -> (NaN/Path/Refnum?=w2111:bool)
            n1671 = Divide(x=w2109, y=1.96) -> (x/y=w2106:dbl)
            n1672 = Compound Arithmetic op=OR(w2112, w2111) -> (w2110:bool)
            n1673 = Not A Number/Path/Refnum?(number/path/refnum=w2106) -> (NaN/Path/Refnum?=w2107:bool)
            n1674 = case shown="True" w2110 {
              frame False {
              }
              frame True {
                n1675 = local write "TEMP"(0.0 ("TEMP")) -> ()
                n1676 = local write "FF 2"(0.0 ("FF 2")) -> ()
                n1677 = local write "reinit"(TRUE ("reinit")) -> ()
              }
            }
            n1678 = local write "TEMP"(w2096) -> ()
            n1679 = Select(t=0.0, s=w2107, f=w2106) -> (s? t:f=w2099:dbl)
            "COF 2" <- w2099
            n1680 = local write "COF 3"(w2099) -> ()
          }
        }
      }
    }
    n1681 = Wait (ms)(milliseconds to wait=u32 50) -> ()  [unwired: 1 out]
    n1682 = local read "Quit"() -> (w2050:bool)
    "Rate" <- 2500.0 ("No of Samples")
  }
  n1683 = while {
    tunnel: [w2140] -> _
    tunnel: [w2123] -> w56
    tunnel: w1 -> [_]
    i -> [w2140]
    stop <- w2123 stop-if-true
    # "C:\\LAB-IQ-NXT\\Scar View.exe"
    n1684 = local read "OK Button 16"() -> (w2130:bool)
    n1685 = local read "Main Tab"() -> (w2124:T2)
    n1686 = local read "service 3"() -> (w2125:bool)
    n1687 = local read "OPEN 6"() -> (w2127:bool)
    n1688 = local read "EDIT 2"() -> (w2129:bool)
    n1689 = flat-sequence {
      frame #0 {
        n1690 = stacked-sequence {
          frame #0 {
            n1691 = local read "EDIT"() -> (w2618:bool)
            n1692 = case shown="False" w2618 {
              tunnel: [u8 2 ("Disabled") u8 0 ("Disabled")] -> _
              frame False {
                w2620 = FALSE
                n1693 = local write "Password"("") -> ()
                n1694 = local write "x = y?"(w2620) -> ()
                n1695 = property on="Password" class="Str"("Visible"=w2620) -> ()  [unwired: 2 in, 2 out]
              }
              frame True {
                n1696 = property on="Password" class="Str"("Visible"=TRUE) -> ()  [unwired: 2 in, 2 out]
              }
            }
            "dipl pwd" <- "@143$\n" ("dipl pwd")
          }
          frame #1 {
          }
          frame #2 {
          }
          frame #3 {
          }
          frame #4 {
            n1697 = String To Byte Array(string="Password") -> (unsigned byte array=w2631:u8[])
            n1698 = Search 1D Array(1D array=w2631, element=u8 10) -> (index of element=w2629:i32)  [unwired: 1 in]
            n1699 = Index Array(array=w2631, index=w2629) -> (element=w2630:u8)
            n1700 = Equal?(x=w2630, y=10) -> (x = y?=w2626:bool)
            n1701 = case shown="True" w2626 {
              frame False {
              }
              frame True {
                # "password"
                # "password"
                n1702 = local read "Password"() -> (w2643:string)
                n1703 = String To Byte Array(string=w2643) -> (unsigned byte array=w2646:u8[])
                n1704 = String To Byte Array(string="@143$\n") -> (unsigned byte array=w2633:u8[])
                n1705 = Array Size(array=w2646) -> (size(s)=w2642:i32)
                n1706 = Array Size(array=w2633) -> (size(s)=w2638:i32)
                n1707 = for {
                  N: w2642 -> [_]
                  tunnel: w2646 -> [w2659]
                  tunnel: [w2657] -> w2647 mode=indexing
                  tunnel: w2642 -> [w2654]
                  i -> [w2655]
                  n1708 = Decrement(x=w2654) -> (x-1=w2653:i32)
                  n1709 = Index Array(array=w2659, index=w2655) -> (element=w2658:u8)
                  n1710 = Equal?(x=w2655, y=w2653) -> (x = y?=w2652:bool)
                  n1711 = Number To Decimal String(number=w2658) -> (decimal integer string=w2656:string)  [unwired: 1 in]
                  n1712 = Select(t="", s=w2652, f="\r") -> (s? t:f=w2649:string)
                  n1713 = Concatenate Strings(w2656, w2649) -> (w2657:string)
                }
                n1714 = for {
                  N: w2638 -> [_]
                  tunnel: w2633 -> [w2670]
                  tunnel: [w2668] -> w2636 mode=indexing
                  tunnel: w2638 -> [w2665]
                  i -> [w2666]
                  n1715 = Decrement(x=w2665) -> (x-1=w2664:i32)
                  n1716 = Index Array(array=w2670, index=w2666) -> (element=w2669:u8)
                  n1717 = Equal?(x=w2666, y=w2664) -> (x = y?=w2663:bool)
                  n1718 = Number To Decimal String(number=w2669) -> (decimal integer string=w2667:string)  [unwired: 1 in]
                  n1719 = Select(t="", s=w2663, f="\r") -> (s? t:f=w2660:string)
                  n1720 = Concatenate Strings(w2667, w2660) -> (w2668:string)
                }
                n1721 = local read "file path"() -> (w2632:path)
                n1722 = call <vilib>:"Read Characters From File.vi"("file path (dialog if empty)"=w2632) -> ("character string"=w2645:string)  [unwired: 5 in, 3 out]
                "string" <- w2645
                n1723 = flat-sequence {
                  tunnel: [w2648] -> _
                  frame #0 {
                    w2648 = ""
                    n1724 = local write "Password"(w2648) -> ()
                  }
                }
                n1725 = Concatenate Strings(w2636) -> (w2637:string)
                n1726 = Concatenate Strings(w2645) -> (w2644:string)
                n1727 = Concatenate Strings(w2647) -> (w2640:string)
                n1728 = Equal?(x=w2640, y=w2644) -> (x = y?=w2635:bool)
                n1729 = Equal?(x=w2640, y=w2637) -> (x = y?=w2641:bool)
                n1730 = Or(x=w2635, y=w2641) -> (x .or. y?=→"x = y?":bool)
              }
            }
          }
        }
        n1731 = local read "x = y?"() -> (w2616:bool)
        n1732 = And(x="EDIT", y=w2616) -> (x .and. y?=w2614:bool)
        n1733 = case shown="True" w2614 {
          tunnel: [u8 2 ("Disabled") u8 0 ("Disabled")] -> w2613
          tunnel: [w2820 TRUE ("Visible")] -> w2612
          frame False {
            w2820 = FALSE ("Visible")
            n1734 = local write "EDIT 2"(w2820) -> ()
          }
          frame True {
          }
        }
        n1735 = case shown="True" "SAVE" {
          frame False {
          }
          frame True {
            n1736 = stacked-sequence {
              seq-local: [w2675 _ _] -> [_ w2816 _]
              frame #0 {
                w2671 = 0.0 ("number")
                w2672 = 0.0 ("number")
                (unwired) i16 5 ("precision (6)")
                # "[CH1]    - FF\n[CH2]   - TEMPERATURE\n[CH3]    - Humidity\n[CH4]    - AIR TEMP\n[CH5]\\- Visa Uno\n[CH6] \\- Visa Due\n[CH7]  \\- file path\n[CH8]   - Displacement Gain\n[CHA]   - Stroke Gain\n[CHB]   - Stroke PID Gain\n[CHC]   -Language Selection\n[CHD]   -Power +\n[CHE]   -Power_\n[CHF]   -Heater\n[CHG]   -Humidity Wet\n[CHH]   -Humidity Dry\n[CHI]   -Integral Time"
                n1737 = local read "Language Selection"() -> (w2718:enum16{"English", "Russian"})
                n1738 = Path To String(path="File Path") -> (string=w2734:string)
                n1739 = Number To Fractional String(number=w2671, width (-)=i16 10 ("precision (6)"), precision (6)=i16 5) -> (F-format string=w2725:string)  [unwired: 1 in]
                n1740 = Number To Fractional String(number=w2718, width (-)=i16 10 ("precision (6)"), precision (6)=i16 5) -> (F-format string=w2714:string)  [unwired: 1 in]
                n1741 = Number To Fractional String(number=w2672, width (-)=i16 10 ("precision (6)"), precision (6)=i16 5) -> (F-format string=w2708:string)  [unwired: 1 in]
                n1742 = Number To Fractional String(number=w2672, width (-)=i16 10 ("precision (6)"), precision (6)=i16 5) -> (F-format string=w2705:string)  [unwired: 1 in]
                n1743 = Number To Fractional String(number=w2672, width (-)=i16 10 ("precision (6)"), precision (6)=i16 5) -> (F-format string=w2700:string)  [unwired: 1 in]
                n1744 = Number To Fractional String(number=w2672, width (-)=i16 10 ("precision (6)"), precision (6)=i16 5) -> (F-format string=w2697:string)  [unwired: 1 in]
                n1745 = Number To Fractional String(number=w2672, width (-)=i16 10 ("precision (6)"), precision (6)=i16 5) -> (F-format string=w2692:string)  [unwired: 1 in]
                n1746 = local read "Com Port 1"() -> (w2674:refnum<visa-resource-name>)
                n1747 = local read "Com Port 2"() -> (w2673:refnum<visa-resource-name>)
                n1748 = Concatenate Strings(w2734, "\\" ("string")) -> (w2733:string)
                n1749 = Number To Fractional String(number=w2671, width (-)=i16 10 ("precision (6)"), precision (6)=i16 5) -> (F-format string=w2766:string)  [unwired: 1 in]
                n1750 = Number To Fractional String(number=w2671, width (-)=i16 10 ("precision (6)"), precision (6)=i16 5) -> (F-format string=w2765:string)  [unwired: 1 in]
                n1751 = Number To Fractional String(number=w2671, width (-)=i16 10 ("precision (6)"), precision (6)=i16 5) -> (F-format string=w2759:string)  [unwired: 1 in]
                n1752 = Number To Fractional String(number=w2671, width (-)=i16 10 ("precision (6)"), precision (6)=i16 5) -> (F-format string=w2753:string)  [unwired: 1 in]
                n1753 = Number To Fractional String(number=w2671, width (-)=i16 10 ("precision (6)"), precision (6)=i16 5) -> (F-format string=w2726:string)  [unwired: 1 in]
                n1754 = Concatenate Strings("[CHA]" ("string"), w2725, "- Stroke Gain" ("string"), "\r") -> (w2719:string)
                n1755 = Concatenate Strings("[CHC]" ("string"), w2714, "-Language Selection" ("string"), "\r") -> (w2711:string)
                n1756 = Concatenate Strings("[CHD]" ("string"), w2708, "-Power +" ("string"), "\r") -> (w2690:string)
                n1757 = Concatenate Strings("[CHG]" ("string"), w2697, "-Humidity Wet" ("string"), "\r") -> (w2687:string)
                n1758 = Concatenate Strings("[CHH]" ("string"), w2692, "-Humidity Dry" ("string"), "\r") -> (w2686:string)
                n1759 = Concatenate Strings("[CH1]" ("string"), w2766, " - FF" ("string"), "\r") -> (w2764:string)
                n1760 = Concatenate Strings("[CH2]" ("string"), w2765, " - TEMPERATURE" ("string"), "\r") -> (w2763:string)
                n1761 = Concatenate Strings("[CH3]" ("string"), w2759, " - Humidity" ("string"), "\r") -> (w2756:string)
                n1762 = Concatenate Strings("[CH4]" ("string"), w2753, " - AIR TEMP" ("string"), "\r") -> (w2749:string)
                n1763 = Concatenate Strings("[CH5]" ("string"), w2674, "- Visa Uno" ("string"), "\r") -> (w2742:string)
                n1764 = Concatenate Strings("[CH6]" ("string"), w2673, "- Visa Due" ("string"), "\r") -> (w2737:string)
                n1765 = Concatenate Strings("[CH7]" ("string"), w2733, "- file path" ("string"), "\r") -> (w2736:string)
                n1766 = Concatenate Strings("[CH8]" ("string"), w2726, "- Displacement Gain" ("string"), "\r") -> (w2729:string)
                n1767 = Concatenate Strings("[CHE]" ("string"), w2705, "-Power_" ("string"), "\r") -> (w2689:string)
                n1768 = Concatenate Strings("[CHF]" ("string"), w2700, "-Heater" ("string"), "\r") -> (w2688:string)
                n1769 = Concatenate Strings(w2764, w2763, w2756, w2749, w2742, w2737, w2736, w2729, w2719, w2711, w2690, w2689, w2688, w2687, w2686) -> (w2675:string)
                "gain" <- w2675
              }
              frame #1 {
                w2777 = 0.0 ("number")
                n1770 = local read "Camera Port :"() -> (w2780:string)
                n1771 = local read "C3 :"() -> (w2788:refnum<visa-resource-name>)
                n1772 = local read "Com Port 3"() -> (w2789:refnum<visa-resource-name>)
                n1773 = Concatenate Strings("[CH8]" ("string"), w2780, "- Visa Camera" ("string"), "\r") -> (w2779:string)
                n1774 = Concatenate Strings("[CH7]" ("string"), w2788, "- Visa Humidity" ("string"), "\r") -> (w2784:string)
                n1775 = Number To Fractional String(number=w2777, width (-)=i16 10 ("precision (6)"), precision (6)=i16 5) -> (F-format string=w2804:string)  [unwired: 1 in]
                n1776 = Concatenate Strings("[CHL]" ("string"), w2789, "- Visa humid" ("string"), "\r") -> (w2792:string)
                n1777 = Number To Fractional String(number=w2777, width (-)=i16 10 ("precision (6)"), precision (6)=i16 5) -> (F-format string=w2811:string)  [unwired: 1 in]
                n1778 = Concatenate Strings("[CHK]" ("string"), w2804, "-TEMP INTERCEPT" ("string"), "\r") -> (w2800:string)
                n1779 = Concatenate Strings("[SNO]" ("string"), "" ("string"), "-" ("string"), "\r") -> (w2797:string)
                n1780 = Concatenate Strings("[CHJ]" ("string"), w2811, "-AIR TEMP INTERCEPT" ("string"), "\r") -> (w2801:string)
                n1781 = String To Path(string="C:\\LAB-IQ\\calibrate WO 2465.dcf") -> (path=w2790:path)
                n1782 = Concatenate Strings(w2816, w2801, w2800, w2797, w2792, w2784, w2779) -> (w2815:string)
                n1783 = call <vilib>:"Write Characters To File.vi"("append to file? (new file:F)"=FALSE, "character string"=w2815, "file path (dialog if empty)"=w2790) -> ()  [unwired: 2 in, 1 out]
              }
              frame #2 {
                n1784 = local write "Lan flag"(0.0 ("Lan flag")) -> ()
                n1785 = local write "conststatus"(0.0 ("rpm value : 2")) -> ()
                n1786 = local write "SAVE"(FALSE ("OK Button 14")) -> ()
              }
            }
          }
        }
        n1787 = property on="EDIT 2" class="Bool (strict)"("Visible"=w2612) -> ()  [unwired: 2 in, 2 out]
        n1788 = property on="SAVE" class="Bool (strict)"("Visible"=w2612) -> ()  [unwired: 2 in, 2 out]
        n1789 = property on="visa due" class="CmbBox"("Disabled"=w2613) -> ()  [unwired: 2 in, 2 out]
        n1790 = property on="File Path" class="Path"("Disabled"=w2613) -> ()  [unwired: 2 in, 2 out]
        n1791 = property on="Language Selection" class="Enum (strict)"("Visible"=w2612) -> ()  [unwired: 2 in, 2 out]
        n1792 = property on="SPEED OUT:" class="DigNum (strict)"("Disabled"=w2613) -> ()  [unwired: 2 in, 2 out]
      }
    }
    n1793 = local read "RUN"() -> (w2139:bool)
    n1794 = local read "RUN"() -> (w2137:bool)
    n1795 = case shown="True" "EDIT 3" {
      frame False {
      }
      frame True {
        n1796 = local write "EDIT 3"(FALSE ("EDIT 3")) -> ()
        n1797 = local write "Main Tab"(T2."About" ("Main Tab")) -> ()
      }
    }
    n1798 = case shown="False" w2139 {
      frame False {
        n1799 = local read "stopT"() -> (w2827:bool)
        n1800 = case shown="True" w2827 {
          frame False {
          }
          frame True {
            n1801 = local write "stopT"(FALSE) -> ()
          }
        }
      }
      frame True {
        "stopT" <- TRUE
      }
    }
    n1802 = case shown="False" w2137 {
      frame False {
      }
      frame True {
      }
    }
    n1803 = case shown="True" w2129 {
      frame False {
        n1804 = property on="Password 2" class="Str"("Visible"=FALSE) -> ()  [unwired: 2 in, 2 out]
        n1805 = local write "Password 2"("" ("Password")) -> ()
      }
      frame True {
        n1806 = property on="Password 2" class="Str"("Visible"=TRUE) -> ()  [unwired: 2 in, 2 out]
        n1807 = Equal?(x="Password 2", y="HFRR1234") -> (x = y?=w2152:bool)
        n1808 = case shown="True" w2152 {
          tunnel: "Password 2" -> [w2155 _]
          frame False {
            n1809 = String Length(string=w2155) -> (length=w2156:i32)
            n1810 = Greater Than 0?(x=w2156) -> (x > 0?=w2154:bool)
            n1811 = case shown="False" w2154 {
              frame False {
                n1812 = property on="Password 2" class="Str"("Caption.Text"="Password (Advance Setting)") -> ()  [unwired: 2 in, 2 out]
              }
              frame True {
                n1813 = property on="Password 2" class="Str"("Caption.Text"="Incorrect Password!") -> ()  [unwired: 2 in, 2 out]
              }
            }
          }
          frame True {
            n1814 = local write "EDIT 2"(FALSE ("EDIT 2")) -> ()
            n1815 = local write "Password 2"("" ("Password")) -> ()
            n1816 = local write "Main Tab"(T2."Advance" ("Main Tab")) -> ()
            n1817 = local write "Main Dashboard Buttons"(T1."Advance" ("Main Dashboard Buttons")) -> ()
          }
        }
      }
    }
    n1818 = case shown="True" "Prog Uno" {
      frame False {
      }
      frame True {
        n1819 = stacked-sequence {
          frame #0 {
            n1820 = Delete(path (use dialog)=path "C:/LAB-IQ-NXT/UNOCOMPILE.bat" ("working directory")) -> ()  [unwired: 4 in, 3 out]
          }
          frame #1 {
            n1821 = local read "Com Port 1"() -> (w2594:refnum<visa-resource-name>)
            n1822 = Concatenate Strings("cmd.exe /c \"mode " ("command line"), w2594, ":1200,n,8,1\"\n" ("command line")) -> (w2599:string)
            n1823 = Concatenate Strings(w2599, "CD\\\nCD WinDucom\navrdude -C avrdude.conf -v -patmega328p -carduino -P" ("command line"), w2594, " -b115200 -D -Uflash:w:UNO_V20.hex:i\n" ("command line"), "\r") -> (w2601:string)
            "STR" <- w2601
            n1824 = call <vilib>:"Write Characters To File.vi"("append to file? (new file:F)"=FALSE, "character string"=w2601, "file path (dialog if empty)"=path "C:/LAB-IQ/UNOCOMPILE.bat" ("working directory")) -> ()  [unwired: 2 in, 1 out]
          }
          frame #2 {
            n1825 = disable-structure shown="Disabled" {
              frame Disabled {
                w2605 = "cmd.exe  /c \"C:\\LAB-IQ-NXT\\UNOCOMPILE.bat\"" ("string")
                n1826 = local write "Prog Uno"(FALSE ("run minimized? (F)")) -> ()
                n1827 = call <vilib>:"System Exec.vi"("expected output size  (4096)"=u32 65535, "run minimized? (F)"=FALSE, "wait until completion? (T)"=TRUE ("run minimized? (F)"), "working directory"=path "C:/LAB-IQ-NXT", "standard input"=w2605, "command line"=w2605) -> ("error out"=w2604:errorcluster, "standard output"=→"String 42":string)  [unwired: 2 in, 2 out]
                "error out 3" <- w2604
                n1828 = flat-sequence {
                  tunnel: w2604 -> [_]
                  frame #0 {
                  }
                }
              }
              frame Enabled {
              }
            }
          }
        }
      }
    }
    n1829 = case shown="\"ISO 12156\"" "TEST STANDARD" {
      frame "ASTM D6079", Default {
        w2574 = 50.0 ("Hz")
        w2575 = 53.0 ("Set Rh")
        w2577 = 1.0 ("Set Strk")
        w2576 = 60.0 ("Set Temp")
        # "astm hide"
        n1830 = local write "NORMAL LOAD"(200.0 ("NORMAL LOAD")) -> ()
        n1831 = local write "Set Strk"(w2577) -> ()
        n1832 = local write "Set Hz"(w2574) -> ()
        n1833 = local write "Set Temp"(w2576) -> ()
        n1834 = local write "Set Rh"(w2575) -> ()
        n1835 = local write "test time"(75.0 ("test time")) -> ()
        n1836 = local write "Set Stroke:"(w2577) -> ()
        n1837 = local write "Set Humidity:"(w2575) -> ()
        n1838 = local write "Set Frequency:"(w2574) -> ()
        n1839 = local write "Set Temperature:"(w2576) -> ()
        "Test Standard" <- "ASTM D6079" ("Test Standard 2")
      }
      frame "ISO 12156" {
        n1840 = local write "Set Strk"(1.0 ("Set Strk")) -> ()
        n1841 = local write "NORMAL LOAD"(200.0 ("NORMAL LOAD")) -> ()
        n1842 = local write "Set Temp"(60.0 ("Set Temp")) -> ()
        n1843 = local write "test time"(75.0 ("test time")) -> ()
        n1844 = local write "Set Hz"(50.0 ("Hz")) -> ()
        n1845 = local write "Set Rh"(53.0 ("Set Rh")) -> ()
      }
      frame "CEC F-096-A-06" {
        n1846 = local write "Set Strk"(1.0 ("Set Strk")) -> ()
        n1847 = local write "NORMAL LOAD"(200.0 ("NORMAL LOAD")) -> ()
        n1848 = local write "Set Temp"(60.0 ("Set Temp")) -> ()
        n1849 = local write "test time"(75.0 ("test time")) -> ()
        n1850 = local write "Set Hz"(50.0 ("Hz")) -> ()
        n1851 = local write "Set Rh"(53.0 ("Set Rh")) -> ()
      }
      frame "Custom" {
      }
    }
    n1852 = Or(x=w2127, y=w2125) -> (x .or. y?=w2126:bool)
    n1853 = case shown="\"About\"" w2124 {
      tunnel: [T26."Acquire" ("Main Tab") T26."Compare Files" ("Main Tab") T26."About" ("Main Tab")] -> w2135
      frame "Acquire", Default {
      }
      frame "Compare Files" {
      }
      frame "About" {
      }
    }
    n1854 = Or(x=w2130, y="OPEN") -> (x .or. y?=w2131:bool)
    n1855 = case shown="True" w2131 {
      tunnel: w2130 -> [_ w2163]
      frame False {
      }
      frame True {
        n1856 = stacked-sequence {
          tunnel: w2163 -> [_ w2230 _ _]
          frame #0 {
            w2179 = "  " ("String 6")
            n1857 = local write "OPEN"(FALSE ("open")) -> ()
            n1858 = local read "string1 2"() -> (w2167:string)
            n1859 = local read "string1 3"() -> (w2166:string)
            n1860 = local read "string1 4"() -> (w2165:string)
            n1861 = property on="OPEN" class="Bool (strict)"("Visible"=FALSE) -> ()  [unwired: 2 in, 2 out]
            n1862 = local write "String 6"(w2179) -> ()
            n1863 = local write "String 7"(w2179) -> ()
            n1864 = local write "String 8"(w2179) -> ()
            n1865 = local write "String 12"(w2179) -> ()
            n1866 = local read "OK Button 16"() -> (w2164:bool)
            n1867 = String To Path(string=w2167) -> (path=w2175:path)
            n1868 = String To Path(string=w2166) -> (path=w2174:path)
            n1869 = String To Path(string=w2165) -> (path=w2173:path)
            n1870 = case shown="True" w2164 {
              tunnel: [w2180 w2181] -> w2168
              frame False {
                n1871 = local read "string1"() -> (w2180:string)
              }
              frame True {
                n1872 = local read "String Indicator 4"() -> (w2181:string)
              }
            }
            n1873 = Open/Create/Replace File "Open File"(file path (use dialog)=w2175) -> (refnum out=w2171:refnum<file>)  [unwired: 5 in, 2 out]
            n1874 = Open/Create/Replace File "Open File"(file path (use dialog)=w2174) -> (refnum out=w2170:refnum<file>)  [unwired: 5 in, 2 out]
            n1875 = Open/Create/Replace File "Open File"(file path (use dialog)=w2173) -> (refnum out=w2169:refnum<file>)  [unwired: 5 in, 2 out]
            n1876 = while {
              tunnel: w2171 -> [w2193]
              i -> [w2189]
              stop <- w2188 continue-if-true
              (unwired) TRUE ("line mode (F)")
              n1877 = Read from Text File "Read File"(file (use dialog)=w2193) -> (text=w2190:string)  [unwired: 3 in, 3 out]
              n1878 = local write "Numeric 11"(w2189) -> ()
              n1879 = String Length(string=w2190) -> (length=w2192:i32)
              n1880 = Greater?(x=w2192, y=1) -> (0:w2188:bool)
            }
            n1881 = while {
              tunnel: w2170 -> [w2199]
              i -> [w2195]
              stop <- w2194 continue-if-true
              (unwired) TRUE ("line mode (F)")
              n1882 = Read from Text File "Read File"(file (use dialog)=w2199) -> (text=w2196:string)  [unwired: 3 in, 3 out]
              n1883 = local write "Numeric 12"(w2195) -> ()
              n1884 = String Length(string=w2196) -> (length=w2198:i32)
              n1885 = Greater?(x=w2198, y=1) -> (0:w2194:bool)
            }
            n1886 = while {
              tunnel: w2169 -> [w2205]
              i -> [w2201]
              stop <- w2200 continue-if-true
              (unwired) TRUE ("line mode (F)")
              n1887 = Read from Text File "Read File"(file (use dialog)=w2205) -> (text=w2202:string)  [unwired: 3 in, 3 out]
              n1888 = local write "Numeric 13"(w2201) -> ()
              n1889 = String Length(string=w2202) -> (length=w2204:i32)
              n1890 = Greater?(x=w2204, y=1) -> (0:w2200:bool)
            }
            n1891 = String To Path(string=w2168) -> (path=w2176:path)
            n1892 = Open/Create/Replace File "Open File"(file path (use dialog)=w2176) -> (refnum out=w2172:refnum<file>)  [unwired: 5 in, 2 out]
            n1893 = while {
              tunnel: w2172 -> [w2187]
              i -> [w2183]
              stop <- w2182 continue-if-true
              (unwired) TRUE ("line mode (F)")
              n1894 = Read from Text File "Read File"(file (use dialog)=w2187) -> (text=w2184:string)  [unwired: 3 in, 3 out]
              n1895 = local write "Numeric 8"(w2183) -> ()
              n1896 = String Length(string=w2184) -> (length=w2186:i32)
              n1897 = Greater?(x=w2186, y=1) -> (0:w2182:bool)
            }
          }
          frame #1 {
            w2357 = FALSE ("ACTUAL   MERGE")
            # "Sample Temp"
            # "ECR"
            # "COF"
            # "Time\nCOF\nFF\nTemp"
            n1898 = case shown="True" w2230 {
              tunnel: [w2377 w2378] -> w2231
              frame False {
